vi "MU generate Biss Identifier.vi"(8 "Error In":errorcluster, 11 "handle":u64) -> (0 "Error Out":errorcluster, 1 "mfgID":u16 format="%.0x", 2 "deviceID":u64 format="%.0x", 3 "function return":u32)   [LabVIEW 2017, in "MU_3SL_interface.lvlib"]
uses:
  MU_3SL_interface.lvlib
  lib/MU_3SL_interface.dll
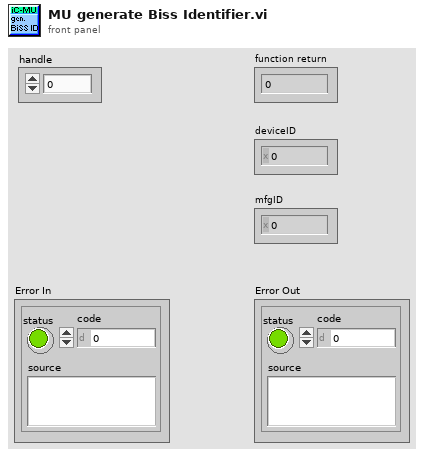
[diagram p1: front panel]
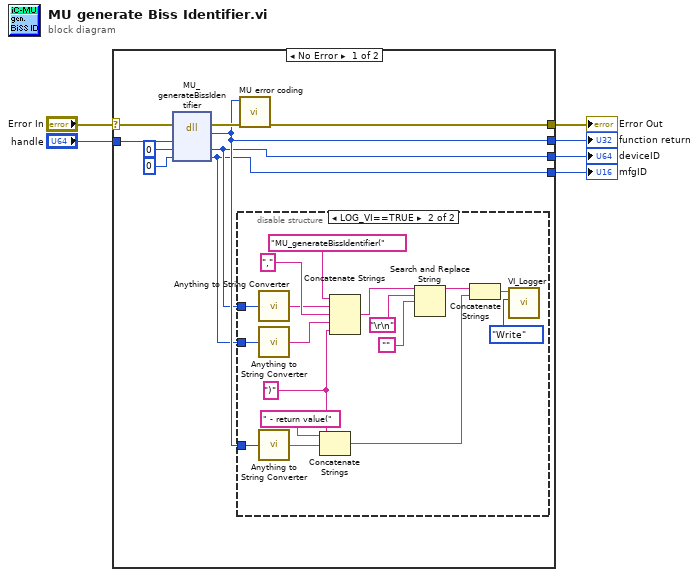
[diagram p0: block diagram]
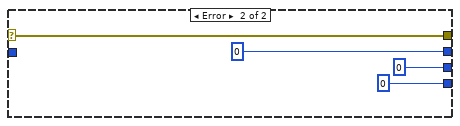
[diagram p3: hidden frame]
diagram:
  n1 = case shown="No Error" "Error In" {
    selector: "Error In" -> [w12 w36]
    tunnel: [w11 u32 0 ("return type")] -> w6
    tunnel: "handle" -> [w15 _]
    tunnel: [w13 w36] -> w4
    tunnel: [w8 u64 0 ("deviceID")] -> w2
    tunnel: [w7 u16 0 ("mfgID")] -> w1
    frame No Error {
      n2 = dll-call lib="C:/Users/bes/AppData/Roaming/work/mu_9so/icsubmodules/soft_mu_3sl_master/lv_interface/lib/MU_3SL_interface**.*" fn="MU_generateBissIdentifier"(error in=w12, "handle"=w15, "deviceID"=u64 0, "mfgID"=u16 0) -> (error out=w14:errorcluster, "return type"=w11:u32, "deviceID"=w8:u64, "mfgID"=w7:u16)  [unwired: 3 in, 1 out]
      n3 = disable-structure shown="LOG_VI==TRUE" {
        disable-tunnel: w11 -> [_ w17]
        disable-tunnel: w8 -> [_ w19]
        disable-tunnel: w7 -> [_ w21]
        frame condition #0 {
        }
        frame condition #1 (active) {
          w27 = ")" ("string")
          n4 = call "Anything to String Converter.vi"("anything"=w19) -> ("String"=w18:string)
          n5 = call "Anything to String Converter.vi"("anything"=w21) -> ("String"=w20:string)
          n6 = call "Anything to String Converter.vi"("anything"=w17) -> ("String"=w16:string)
          n7 = Concatenate Strings(" - return value(" ("string"), w16, w27) -> (w30:string)
          n8 = Concatenate Strings("MU_generateBissIdentifier(" ("Info in"), w18, "," ("string"), w20, w27) -> (w24:string)
          n9 = Search and Replace String(input string=w24, search string="\r\n", replace string="") -> (result string=w23:string)  [unwired: 5 in, 3 out]
          n10 = Concatenate Strings(w23, w30) -> (w29:string)
          n11 = call "VI_Logger.vi"("Action (Read)"=enum16{"Write", "Read"}."Write", "Info in"=w29) -> ()  [unwired: 8 in, 2 out]
        }
      }
      n12 = call "MU error coding.vi"("error in (no error)"=w14, "function return in"=w11) -> ("error out"=w13:errorcluster)  [unwired: 9 in]
    }
    frame Error {
    }
  }
  "function return" <- w6
  "Error Out" <- w4
  "mfgID" <- w1
  "deviceID" <- w2
